vi "Write Measurement Interval Refnum.vi"(8 "error in (no error)":errorcluster, 10 "Measurement Interval Refnum":refnum<vi>, 11 "Generic Card in":refnum<class "Generic Card.lvclass">) -> (0 "error out":errorcluster, 3 "Generic Card out":refnum<class "Generic Card.lvclass">)   [LabVIEW 2012]
uses:
  Generic Card.lvclass
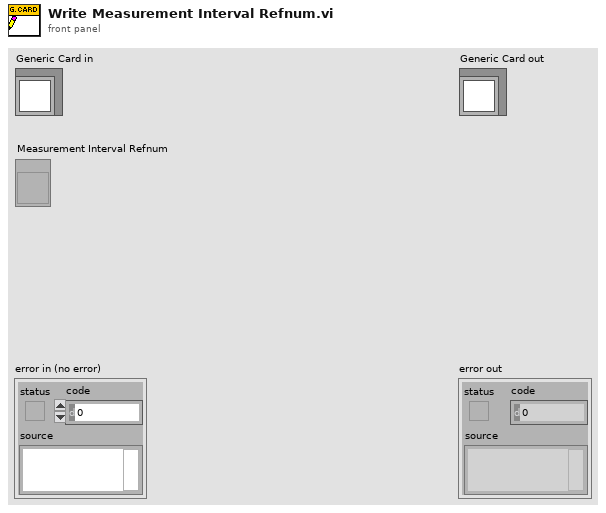
[diagram p1: front panel]
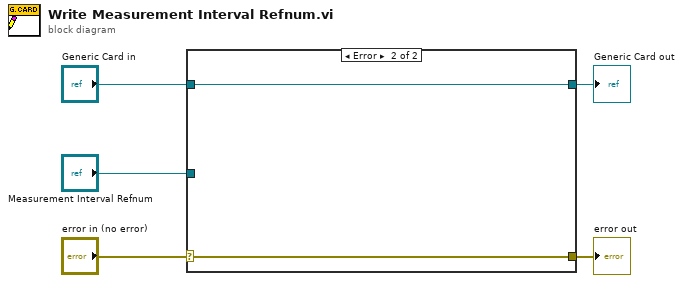
[diagram p0: block diagram]
diagram:
  n1 = case shown="Error" "error in (no error)" {
    selector: "error in (no error)" -> [w7 w8]
    tunnel: [w7 w8] -> w4
    tunnel: [w6 w9] -> w2
    tunnel: "Generic Card in" -> [w6 w9]
    tunnel: "Measurement Interval Refnum" -> [_ _]
    frame No Error {
    }
    frame Error {
    }
  }
  "error out" <- w4
  "Generic Card out" <- w2
